vi "Fpga-U64-U8-Array.vi"(11 "U64 in":u64) -> (3 "U8[] out":u8[](array[numeric]))   [LabVIEW 2018]
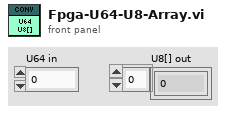
[diagram p1: front panel]
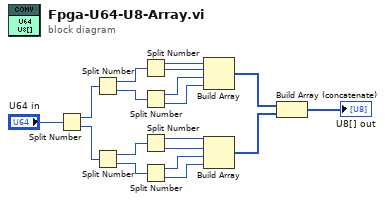
[diagram p0: block diagram]
diagram:
  n1 = Split Number(x="U64 in") -> (hi(x)=w1:u32, lo(x)=w2:u32)
  n2 = Split Number(x=w1) -> (hi(x)=w6:u16, lo(x)=w5:u16)
  n3 = Split Number(x=w2) -> (hi(x)=w4:u16, lo(x)=w3:u16)
  n4 = Split Number(x=w6) -> (hi(x)=w8:u8, lo(x)=w9:u8)
  n5 = Split Number(x=w5) -> (hi(x)=w10:u8, lo(x)=w11:u8)
  n6 = Split Number(x=w4) -> (hi(x)=w12:u8, lo(x)=w13:u8)
  n7 = Split Number(x=w3) -> (hi(x)=w14:u8, lo(x)=w15:u8)
  n8 = Build Array(w8, w9, w10, w11) -> (w16:u8[])
  n9 = Build Array(w12, w13, w14, w15) -> (w17:u8[])
  n10 = Build Array (concatenate)(w16, w17) -> (→"U8[] out":u8[])
